vi "Protect Against Broken Encoders.vi"(3 "Encoder Input":dbl) -> (0 "Broken":bool, 1 "Output":dbl)   [LabVIEW 2019]
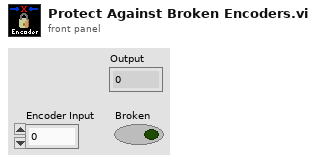
[diagram p1: front panel]
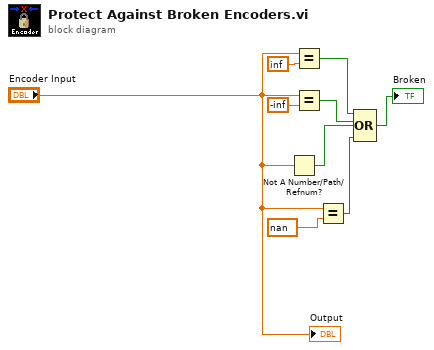
[diagram p0: block diagram]
diagram:
  n1 = Not A Number/Path/Refnum?(number/path/refnum="Encoder Input") -> (NaN/Path/Refnum?=w4:bool)
  n2 = Equal?(x="Encoder Input", y=inf) -> (x = y?=w7:bool)
  n3 = Equal?(x="Encoder Input", y=-inf) -> (x = y?=w6:bool)
  n4 = Equal?(x="Encoder Input", y=nan) -> (x = y?=w2:bool)
  n5 = Compound Arithmetic op=OR(w7, w6, w4, w2) -> (→"Broken":bool)
  "Output" <- "Encoder Input"
